vi "Autonomous Independent.vi"   [LabVIEW 2020]
doc: "This VI is called when autonomous begins, and will automatically be terminated when autonomous ends. You can carry out timed or sensor driven robot movement independently without needing to return to the caller."
uses:
  <vilib>/Rock Robotics/Network Tables/NT Read String.vi
  Robot Global Data.vi
panel:
  # "Be sure to right-click and choose Data Operations>>Make Current Value default if you want to save the array values with the VI"
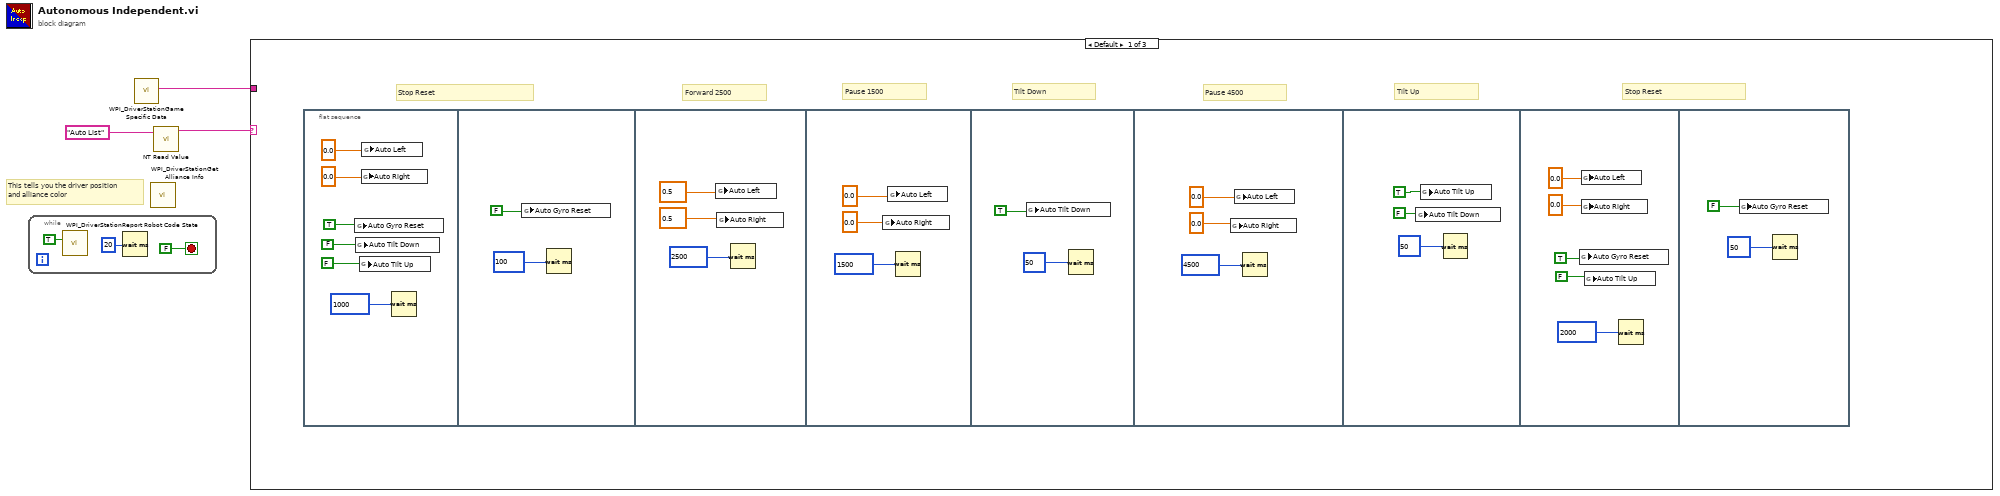
[diagram p0: block diagram]
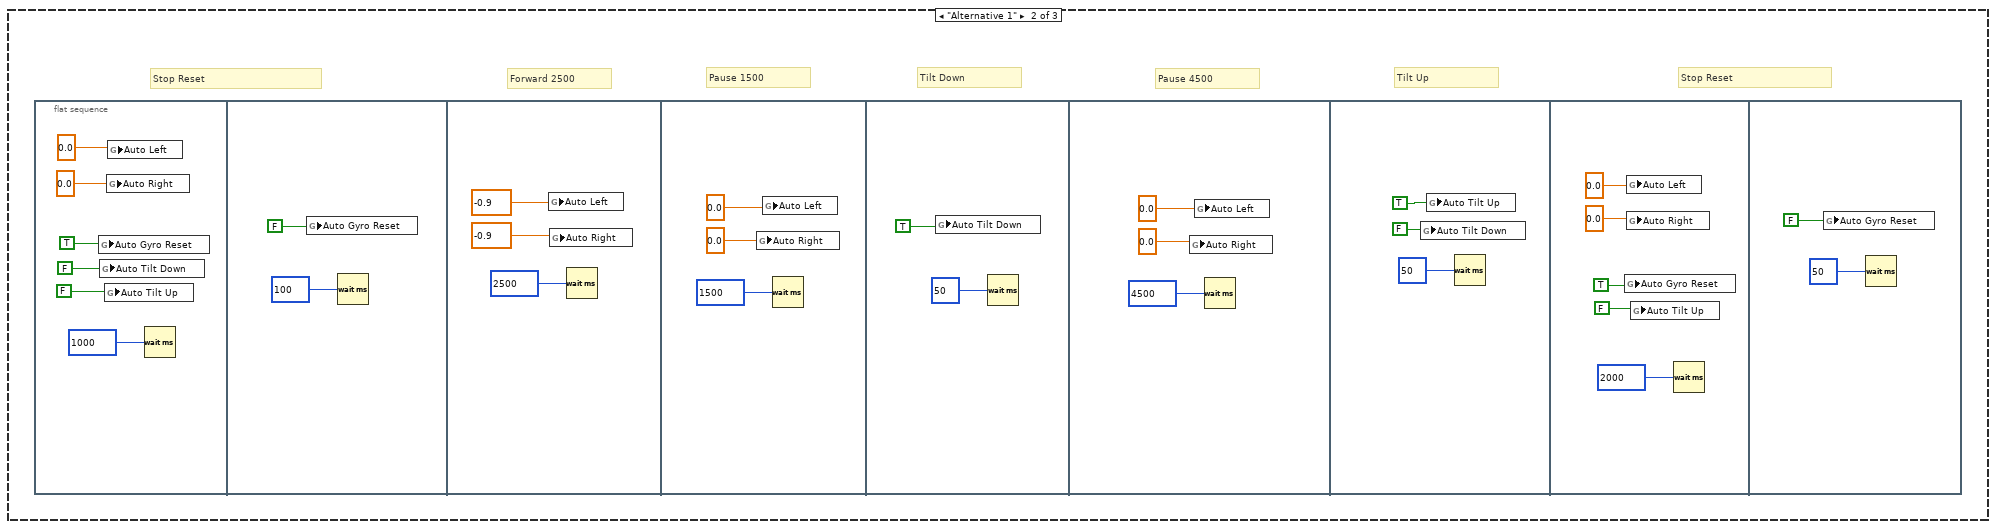
[diagram p2: hidden frame]
diagram:
  # "This tells you the driver position\nand alliance color"
  n1 = while {
    stop <- FALSE stop-if-true
    n2 = call <vilib>:"WPI_DriverStationReport Robot Code State.vi"("Autonomous"=TRUE) -> ()  [unwired: 10 in, 1 out]
    n3 = Wait (ms)(milliseconds to wait=u32 20) -> ()  [unwired: 1 out]
  }
  n4 = call <vilib>:"WPI_DriverStationGame Specific Data.vi"() -> ("Game Specific Data"=w1:string)  [unwired: 11 in]
  n5 = call <vilib>:"WPI_DriverStationGet Alliance Info.vi"() -> ()  [unwired: 12 out]
  n6 = call-poly <vilib>:"NT Read Value.vi"("Name"="Auto List") -> ("String"=w2:string)  [unwired: 9 in, 1 out]
  n7 = case shown="Default" w2 {
    tunnel: w1 -> [_ _ _]
    frame Default {
      # "Stop Reset"
      # "Tilt Up"
      # "Pause 4500"
      # "Tilt Down"
      # "Pause 1500"
      # "Forward 2500"
      # "Stop Reset"
      n8 = flat-sequence {
        frame #0 {
          n9 = global write "Robot Global Data.vi" "Auto Gyro Reset"(TRUE) -> ()
          n10 = global write "Robot Global Data.vi" "Auto Tilt Down"(FALSE) -> ()
          n11 = global write "Robot Global Data.vi" "Auto Tilt Up"(FALSE) -> ()
          n12 = global write "Robot Global Data.vi" "Auto Right"(0.0 ("Autonomous Shooter")) -> ()
          n13 = global write "Robot Global Data.vi" "Auto Left"(0.0 ("Autonomous Shooter")) -> ()
          n14 = Wait (ms)(milliseconds to wait=u32 1000) -> ()  [unwired: 1 out]
        }
        frame #1 {
          n15 = global write "Robot Global Data.vi" "Auto Gyro Reset"(FALSE) -> ()
          n16 = Wait (ms)(milliseconds to wait=u32 100) -> ()  [unwired: 1 out]
        }
        frame #2 {
          n17 = global write "Robot Global Data.vi" "Auto Left"(0.5 ("Autonomous Shooter")) -> ()
          n18 = global write "Robot Global Data.vi" "Auto Right"(0.5 ("Autonomous Shooter")) -> ()
          n19 = Wait (ms)(milliseconds to wait=u32 2500) -> ()  [unwired: 1 out]
        }
        frame #3 {
          n20 = global write "Robot Global Data.vi" "Auto Right"(0.0 ("Autonomous Shooter")) -> ()
          n21 = global write "Robot Global Data.vi" "Auto Left"(0.0 ("Autonomous Shooter")) -> ()
          n22 = Wait (ms)(milliseconds to wait=u32 1500) -> ()  [unwired: 1 out]
        }
        frame #4 {
          n23 = global write "Robot Global Data.vi" "Auto Tilt Down"(TRUE) -> ()
          n24 = Wait (ms)(milliseconds to wait=u32 50) -> ()  [unwired: 1 out]
        }
        frame #5 {
          n25 = global write "Robot Global Data.vi" "Auto Right"(0.0 ("Autonomous Shooter")) -> ()
          n26 = global write "Robot Global Data.vi" "Auto Left"(0.0 ("Autonomous Shooter")) -> ()
          n27 = Wait (ms)(milliseconds to wait=u32 4500) -> ()  [unwired: 1 out]
        }
        frame #6 {
          n28 = global write "Robot Global Data.vi" "Auto Tilt Down"(FALSE) -> ()
          n29 = global write "Robot Global Data.vi" "Auto Tilt Up"(TRUE) -> ()
          n30 = Wait (ms)(milliseconds to wait=u32 50) -> ()  [unwired: 1 out]
        }
        frame #7 {
          n31 = global write "Robot Global Data.vi" "Auto Gyro Reset"(TRUE) -> ()
          n32 = global write "Robot Global Data.vi" "Auto Left"(0.0 ("Autonomous Shooter")) -> ()
          n33 = global write "Robot Global Data.vi" "Auto Right"(0.0 ("Autonomous Shooter")) -> ()
          n34 = global write "Robot Global Data.vi" "Auto Tilt Up"(FALSE) -> ()
          n35 = Wait (ms)(milliseconds to wait=u32 2000) -> ()  [unwired: 1 out]
        }
        frame #8 {
          n36 = global write "Robot Global Data.vi" "Auto Gyro Reset"(FALSE) -> ()
          n37 = Wait (ms)(milliseconds to wait=u32 50) -> ()  [unwired: 1 out]
        }
      }
    }
    frame "Alternative 1" {
      # "Stop Reset"
      # "Tilt Up"
      # "Pause 4500"
      # "Tilt Down"
      # "Pause 1500"
      # "Forward 2500"
      # "Stop Reset"
      n38 = flat-sequence {
        frame #0 {
          n39 = global write "Robot Global Data.vi" "Auto Gyro Reset"(TRUE) -> ()
          n40 = global write "Robot Global Data.vi" "Auto Tilt Down"(FALSE) -> ()
          n41 = global write "Robot Global Data.vi" "Auto Tilt Up"(FALSE) -> ()
          n42 = global write "Robot Global Data.vi" "Auto Right"(0.0 ("Autonomous Shooter")) -> ()
          n43 = global write "Robot Global Data.vi" "Auto Left"(0.0 ("Autonomous Shooter")) -> ()
          n44 = Wait (ms)(milliseconds to wait=u32 1000) -> ()  [unwired: 1 out]
        }
        frame #1 {
          n45 = global write "Robot Global Data.vi" "Auto Gyro Reset"(FALSE) -> ()
          n46 = Wait (ms)(milliseconds to wait=u32 100) -> ()  [unwired: 1 out]
        }
        frame #2 {
          n47 = global write "Robot Global Data.vi" "Auto Left"(-0.9 ("Autonomous Shooter")) -> ()
          n48 = global write "Robot Global Data.vi" "Auto Right"(-0.9 ("Autonomous Shooter")) -> ()
          n49 = Wait (ms)(milliseconds to wait=u32 2500) -> ()  [unwired: 1 out]
        }
        frame #3 {
          n50 = global write "Robot Global Data.vi" "Auto Right"(0.0 ("Autonomous Shooter")) -> ()
          n51 = global write "Robot Global Data.vi" "Auto Left"(0.0 ("Autonomous Shooter")) -> ()
          n52 = Wait (ms)(milliseconds to wait=u32 1500) -> ()  [unwired: 1 out]
        }
        frame #4 {
          n53 = global write "Robot Global Data.vi" "Auto Tilt Down"(TRUE) -> ()
          n54 = Wait (ms)(milliseconds to wait=u32 50) -> ()  [unwired: 1 out]
        }
        frame #5 {
          n55 = global write "Robot Global Data.vi" "Auto Right"(0.0 ("Autonomous Shooter")) -> ()
          n56 = global write "Robot Global Data.vi" "Auto Left"(0.0 ("Autonomous Shooter")) -> ()
          n57 = Wait (ms)(milliseconds to wait=u32 4500) -> ()  [unwired: 1 out]
        }
        frame #6 {
          n58 = global write "Robot Global Data.vi" "Auto Tilt Down"(FALSE) -> ()
          n59 = global write "Robot Global Data.vi" "Auto Tilt Up"(TRUE) -> ()
          n60 = Wait (ms)(milliseconds to wait=u32 50) -> ()  [unwired: 1 out]
        }
        frame #7 {
          n61 = global write "Robot Global Data.vi" "Auto Gyro Reset"(TRUE) -> ()
          n62 = global write "Robot Global Data.vi" "Auto Left"(0.0 ("Autonomous Shooter")) -> ()
          n63 = global write "Robot Global Data.vi" "Auto Right"(0.0 ("Autonomous Shooter")) -> ()
          n64 = global write "Robot Global Data.vi" "Auto Tilt Up"(FALSE) -> ()
          n65 = Wait (ms)(milliseconds to wait=u32 2000) -> ()  [unwired: 1 out]
        }
        frame #8 {
          n66 = global write "Robot Global Data.vi" "Auto Gyro Reset"(FALSE) -> ()
          n67 = Wait (ms)(milliseconds to wait=u32 50) -> ()  [unwired: 1 out]
        }
      }
    }
    frame "Alternative 2" {
    }
  }
